vi "Teleop.vi"(10 "Match Info":T2={"Autonomous Elapsed Seconds"=0.0, "TeleOp Elapsed Seconds"=0.0, "Disabled Elapsed Seconds"=0.0, "Visited Autonomous"=FALSE, "Visited TeleOp"=FALSE, "Visited Disabled"=FALSE, "Autonomous Settings"={"Autonomous Style"=enum."Independent", "VI Refnum"=refnum}}, 11 "Call Context":T3) -> ()   [LabVIEW 2016]
doc: "This VI is called for each TeleOp packet received from the DS where the robot is not disabled. It is often used to read from the joysticks and update I/O or to update setpoints for timed control loops. It should complete and return within 20 milliseconds or it may miss DS packets."
uses:
  <vilib>/Rock Robotics/WPI/DriverStation/WPI_DriverStationDerivedRobotMode.ctl
  <vilib>/Rock Robotics/WPI/DriverStation/WPI_DriverStationMatch Info.ctl
  Robot Global Data.vi
  <vilib>/Rock Robotics/WPI/Utilities/WPI_GetSetVariantRefNum.vi
  <vilib>/addons/control/pid/pid.llb/PID (DBL).vi
  <vilib>/addons/control/pid/NI_PID_pid.lvlib
panel:
  in  "output range":cluster{"output high":dbl, "output low":dbl}={"output high"=100.0, "output low"=-100.0} {"output low" format="%.2f"; "output high" format="%.2f"}
  in  "PID gains":T1={"proportional gain (Kc)"=1.0, "integral time (Ti, min)"=0.01, "derivative time (Td, min)"=0.0} {"derivative time (Td, min)" format="%.3f"; "integral time (Ti, min)" format="%.3f"; "proportional gain (Kc)" format="%.3f"}
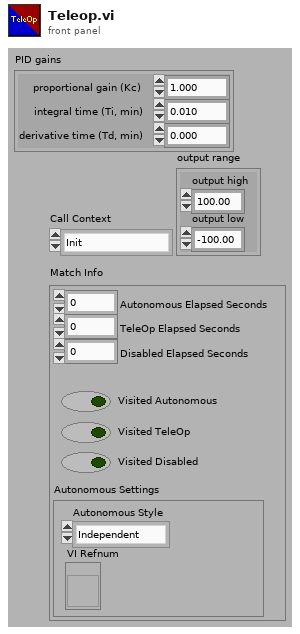
[diagram p1: front panel]
types:
  T1 = cluster{"proportional gain (Kc)":dbl, "integral time (Ti, min)":dbl, "derivative time (Td, min)":dbl}
  T2 = typedef "WPI_DriverStationMatch Info.ctl" = cluster{"Autonomous Elapsed Seconds":dbl, "TeleOp Elapsed Seconds":dbl, "Disabled Elapsed Seconds":dbl, "Visited Autonomous":bool, "Visited TeleOp":bool, "Visited Disabled":bool, "Autonomous Settings":cluster{"Autonomous Style":enum16{"Iterative", "Independent"}, "VI Refnum":refnum<vi>}}
  T3 = typedef "WPI_DriverStationDerivedRobotMode.ctl" = enum16{"Init", "Execute", "Stop"}
  T4 = typedef "WPI_RobotDriveDevRef.ctl" = cluster{"DevStatus":errorcluster, "Motors[]":T5[], "Square Inputs":bool, "Max Output":dbl}
  T5 = typedef "WPI_MotorControlDeviceRef.ctl" = cluster{"DeviceStatus":errorcluster, "Type":T6, "PWM":cluster{"PWM Channel":T7, "DeadBand":T8}, "CAN":cluster{"Device Number":u8, "SetOutput VI Ref":variant, "GetOutput VI Ref":variant, "Enable VI Ref":variant, "Disable VI Ref":variant, "Data":variant}, "Invert":bool}
  T6 = typedef "WPI_MotorControlType.ctl" = enum16{"PWM", "CAN"}
  T7 = typedef "FPGA_DIOPWMChannel.ctl" = enum8{"PWM 0", "PWM 1", "PWM 2", "PWM 3", "PWM 4", "PWM 5", "PWM 6", "PWM 7", "PWM 8", "PWM 9", "PWM MXP 0", "PWM MXP 1", "PWM MXP 2", "PWM MXP 3", "PWM MXP 4", "PWM MXP 5", "PWM MXP 6", "PWM MXP 7", "PWM MXP 8", "PWM MXP 9", "Invalid"}
  T8 = typedef "WPI_PWMDeadband.ctl" = cluster{"Name":string, "maxPositivePwm":i32, "minPositivePwm":i32, "centerPwm":i32, "maxNegativePwm":i32, "minNegativePwm":i32, "angularRange":u16}
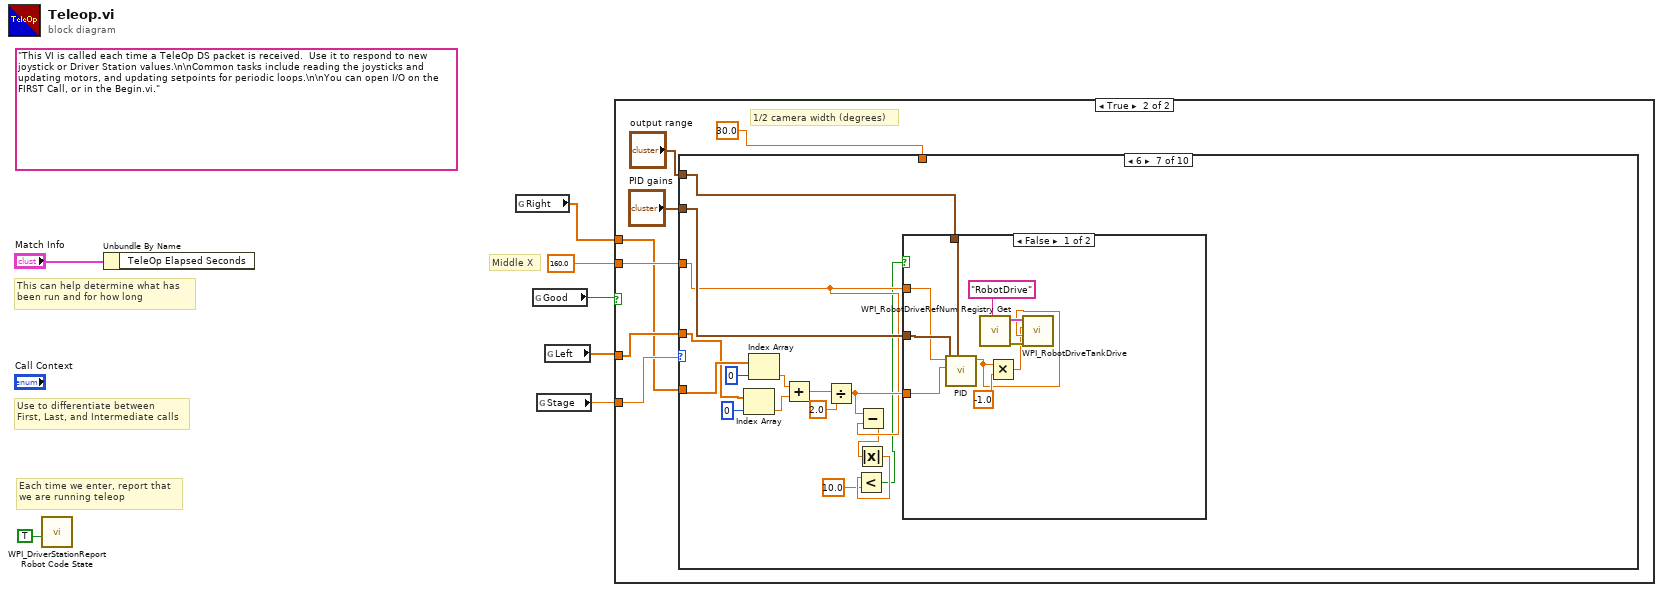
[diagram p0: block diagram]
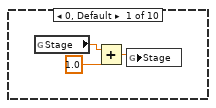
[diagram p3: hidden frame]
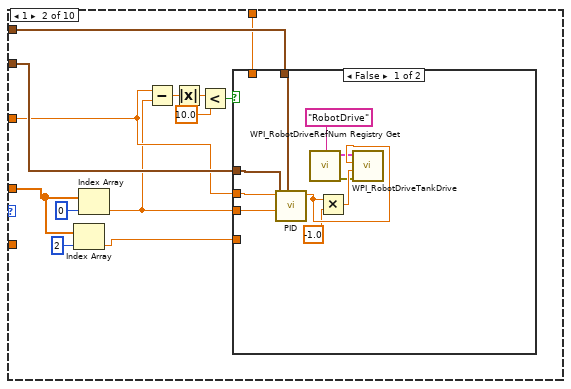
[diagram p4: hidden frame]
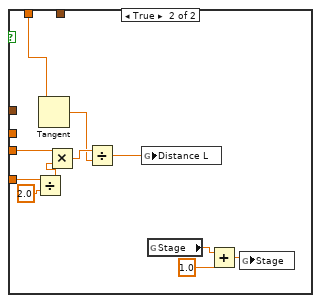
[diagram p5: hidden frame]
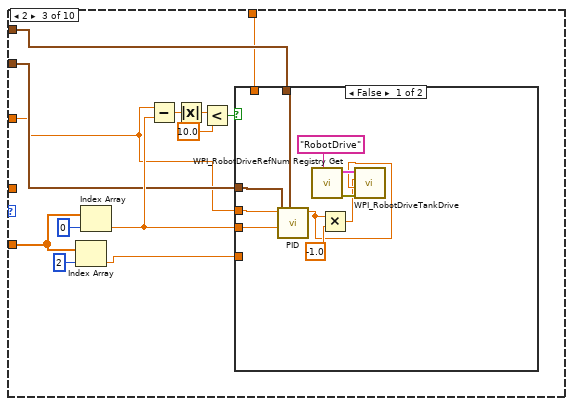
[diagram p6: hidden frame]
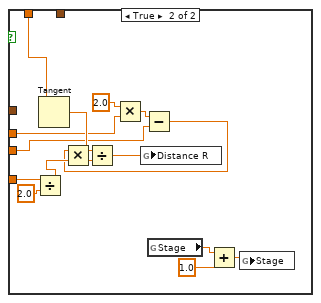
[diagram p7: hidden frame]
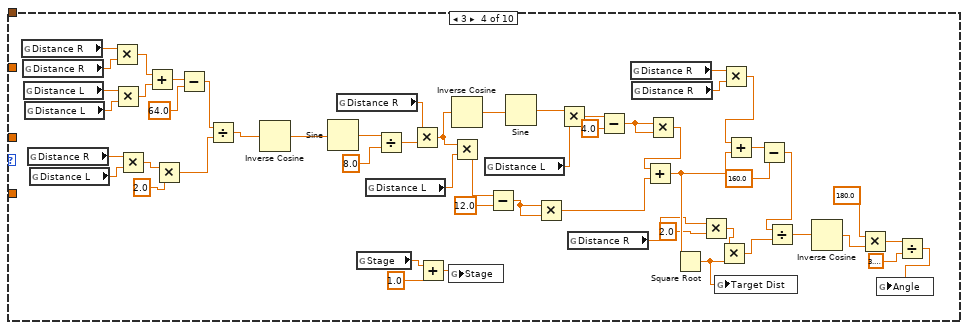
[diagram p8: hidden frame]
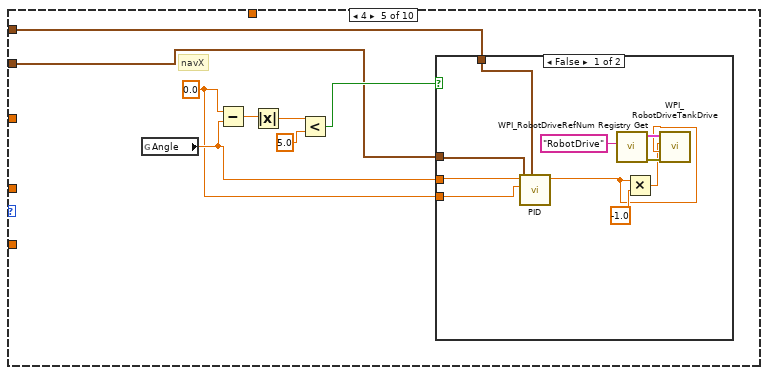
[diagram p9: hidden frame]
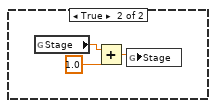
[diagram p10: hidden frame]
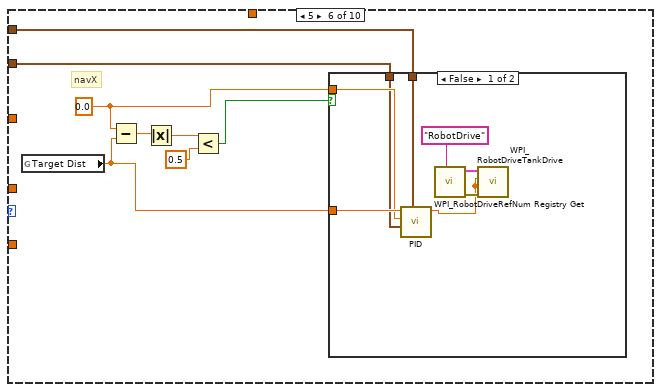
[diagram p11: hidden frame]
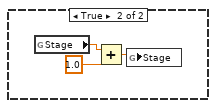
[diagram p12: hidden frame]
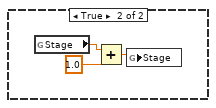
[diagram p13: hidden frame]
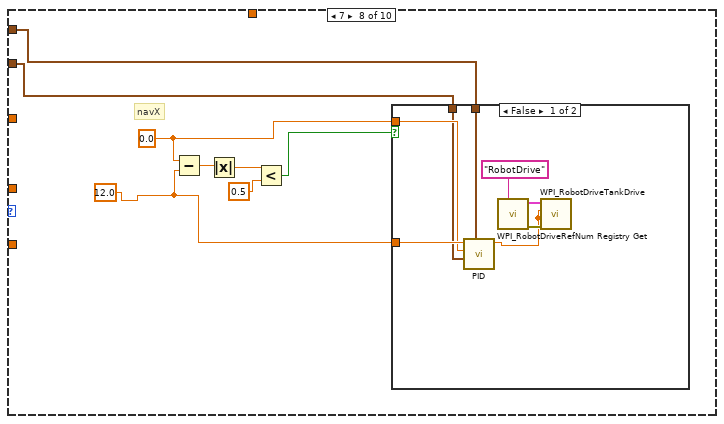
[diagram p14: hidden frame]
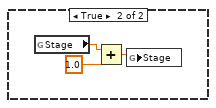
[diagram p15: hidden frame]
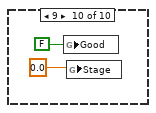
[diagram p17: hidden frame]
diagram:
  (unwired) "This VI is called each time a TeleOp DS packet is received.  Use it to respond to new joystick or Driver Station values.\n\nCommon tasks include reading the joysticks and updating motors, and updating setpoints for periodic loops.\n\nYou can open I/O on the FIRST Call, or in the Begin.vi."
  # "Middle X"
  # "Each time we enter, report that\nwe are running teleop"
  # "Use to differentiate between\nFirst, Last, and Intermediate calls"
  # "This can help determine what has\nbeen run and for how long"
  n1 = call <vilib>:"WPI_DriverStationReport Robot Code State.vi"("TeleOp"=TRUE ("Autonomous")) -> ()  [unwired: 10 in, 1 out]
  n2 = Unbundle By Name("Match Info") -> ()  [unwired: 1 out]
  n3 = global read "Robot Global Data.vi" "Right"() -> (w4:dbl[])
  n4 = global read "Robot Global Data.vi" "Good"() -> (w3:bool)
  n5 = global read "Robot Global Data.vi" "Stage"() -> (w2:dbl)
  n6 = global read "Robot Global Data.vi" "Left"() -> (w5:dbl[])
  n7 = case shown="True" w3 {
    tunnel: w4 -> [_ w8]
    tunnel: w5 -> [_ w13]
    tunnel: w2 -> [_ w14]
    tunnel: 160.0 ("setpoint") -> [_ w12]
    frame False {
    }
    frame True {
      # "1/2 camera width (degrees)"
      n8 = case shown="6" w14 {
        tunnel: w13 -> [_ w20 _ _ _ _ w194 _ _ _]
        tunnel: w12 -> [_ w27 w54 _ _ _ w188 _ _ _]
        tunnel: "PID gains" -> [_ w29 w55 _ w145 w166 w196 w215 _ _]
        tunnel: "output range" -> [_ w28 w56 _ w144 w165 w195 w214 _ _]
        tunnel: 30.0 -> [_ w21 w52 _ _ _ _ _ _ _]
        tunnel: w8 -> [_ _ w53 _ _ _ w197 _ _ _]
        frame 0, Default {
          n9 = global read "Robot Global Data.vi" "Stage"() -> (w17:dbl)
          n10 = Add(x=w17, y=1.0) -> (x+y=w15:dbl)
          n11 = global write "Robot Global Data.vi" "Stage"(w15) -> ()
        }
        frame 1 {
          n12 = Index Array(array=w20, index=2) -> (element=w18:dbl)
          n13 = Index Array(array=w20, index=0) -> (element=w26:dbl)
          n14 = Subtract(x=w27, y=w26) -> (x-y=w25:dbl)
          n15 = Absolute Value(x=w25) -> (abs(x)=w24:dbl)
          n16 = Less?(x=w24, y=10.0) -> (x < y?=w22:bool)
          n17 = case shown="False" w22 {
            tunnel: w29 -> [w34 _]
            tunnel: w28 -> [w35 _]
            tunnel: w27 -> [w33 _]
            tunnel: w26 -> [w32 w45]
            tunnel: w21 -> [_ w48]
            tunnel: w18 -> [_ w47]
            frame False {
              n18 = call-poly <vilib>:"PID.vi"("output range"=w35, "PID gains"=w34, "process variable"=w32, "setpoint"=w33) -> ("output"=w40:dbl)  [unwired: 6 in, 1 out]
              n19 = call <vilib>:"WPI_RobotDriveRefNum Registry Get.vi"("refnum name"="RobotDrive") -> ("error out"=w36:errorcluster, "RobotDriveDevRef"=w37:T4)  [unwired: 9 in]
              n20 = Multiply(x=w40, y=-1.0) -> (x*y=w39:dbl)
              n21 = call <vilib>:"WPI_RobotDriveTankDrive.vi"("error in (no error)"=w36, "Right axis value"=w39, "Left axis value"=w40, "RobotDriveDevRef"=w37) -> ()  [unwired: 5 in, 3 out]
            }
            frame True {
              n22 = Divide(x=w47, y=2.0) -> (x/y=w44:dbl)
              n23 = Tangent(1:w48) -> (0:w42:dbl)
              n24 = Multiply(x=w45, y=w44) -> (x*y=w43:dbl)
              n25 = Divide(x=w43, y=w42) -> (x/y=w41:dbl)
              n26 = global write "Robot Global Data.vi" "Distance L"(w41) -> ()
              n27 = global read "Robot Global Data.vi" "Stage"() -> (w51:dbl)
              n28 = Add(x=w51, y=1.0) -> (x+y=w49:dbl)
              n29 = global write "Robot Global Data.vi" "Stage"(w49) -> ()
            }
          }
        }
        frame 2 {
          n30 = Index Array(array=w53, index=2) -> (element=w57:dbl)
          n31 = Index Array(array=w53, index=0) -> (element=w63:dbl)
          n32 = Subtract(x=w54, y=w63) -> (x-y=w62:dbl)
          n33 = Absolute Value(x=w62) -> (abs(x)=w61:dbl)
          n34 = Less?(x=w61, y=10.0) -> (x < y?=w59:bool)
          n35 = case shown="False" w59 {
            tunnel: w55 -> [w70 _]
            tunnel: w56 -> [w71 _]
            tunnel: w54 -> [w69 w76]
            tunnel: w63 -> [w68 w77]
            tunnel: w52 -> [_ w86]
            tunnel: w57 -> [_ w85]
            frame False {
              n36 = call-poly <vilib>:"PID.vi"("output range"=w71, "PID gains"=w70, "process variable"=w68, "setpoint"=w69) -> ("output"=w67:dbl)  [unwired: 6 in, 1 out]
              n37 = call <vilib>:"WPI_RobotDriveRefNum Registry Get.vi"("refnum name"="RobotDrive") -> ("error out"=w72:errorcluster, "RobotDriveDevRef"=w73:T4)  [unwired: 9 in]
              n38 = Multiply(x=w67, y=-1.0) -> (x*y=w66:dbl)
              n39 = call <vilib>:"WPI_RobotDriveTankDrive.vi"("error in (no error)"=w72, "Right axis value"=w67, "Left axis value"=w66, "RobotDriveDevRef"=w73) -> ()  [unwired: 5 in, 3 out]
            }
            frame True {
              n40 = Divide(x=w85, y=2.0) -> (x/y=w83:dbl)
              n41 = Tangent(1:w86) -> (0:w81:dbl)
              n42 = Multiply(x=2.0, y=w76) -> (x*y=w78:dbl)
              n43 = Subtract(x=w78, y=w77) -> (x-y=w75:dbl)
              n44 = Multiply(x=w75, y=w83) -> (x*y=w82:dbl)
              n45 = Divide(x=w82, y=w81) -> (x/y=w80:dbl)
              n46 = global write "Robot Global Data.vi" "Distance R"(w80) -> ()
              n47 = global read "Robot Global Data.vi" "Stage"() -> (w89:dbl)
              n48 = Add(x=w89, y=1.0) -> (x+y=w87:dbl)
              n49 = global write "Robot Global Data.vi" "Stage"(w87) -> ()
            }
          }
        }
        frame 3 {
          n50 = global read "Robot Global Data.vi" "Distance R"() -> (w143:dbl)
          n51 = global read "Robot Global Data.vi" "Distance R"() -> (w142:dbl)
          n52 = global read "Robot Global Data.vi" "Distance L"() -> (w141:dbl)
          n53 = global read "Robot Global Data.vi" "Distance L"() -> (w140:dbl)
          n54 = global read "Robot Global Data.vi" "Distance R"() -> (w135:dbl)
          n55 = global read "Robot Global Data.vi" "Distance L"() -> (w134:dbl)
          n56 = Multiply(x=w143, y=w142) -> (x*y=w138:dbl)
          n57 = Multiply(x=w141, y=w140) -> (x*y=w139:dbl)
          n58 = Multiply(x=w135, y=w134) -> (x*y=w133:dbl)
          n59 = Add(x=w138, y=w139) -> (x+y=w137:dbl)
          n60 = Multiply(x=w133, y=2.0) -> (x*y=w130:dbl)
          n61 = Subtract(x=w137, y=64.0) -> (x-y=w131:dbl)
          n62 = Divide(x=w131, y=w130) -> (x/y=w129:dbl)
          n63 = Inverse Cosine(1:w129) -> (0:w128:dbl)
          n64 = Sine(x=w128) -> (sin(x)=w127:dbl)
          n65 = global read "Robot Global Data.vi" "Distance R"() -> (w124:dbl)
          n66 = global read "Robot Global Data.vi" "Stage"() -> (w92:dbl)
          n67 = global read "Robot Global Data.vi" "Distance L"() -> (w123:dbl)
          n68 = Divide(x=w127, y=8.0) -> (x/y=w125:dbl)
          n69 = Multiply(x=w124, y=w125) -> (x*y=w122:dbl)
          n70 = Add(x=w92, y=1.0) -> (x+y=w90:dbl)
          n71 = global write "Robot Global Data.vi" "Stage"(w90) -> ()
          n72 = Inverse Cosine(1:w122) -> (0:w121:dbl)
          n73 = Multiply(x=w122, y=w123) -> (x*y=w118:dbl)
          n74 = global read "Robot Global Data.vi" "Distance L"() -> (w119:dbl)
          n75 = Subtract(x=w118, y=12.0) -> (x-y=w114:dbl)
          n76 = Sine(x=w121) -> (sin(x)=w120:dbl)
          n77 = Multiply(x=w114, y=w114) -> (x*y=w111:dbl)
          n78 = Multiply(x=w120, y=w119) -> (x*y=w116:dbl)
          n79 = global read "Robot Global Data.vi" "Distance R"() -> (w102:dbl)
          n80 = Subtract(x=w116, y=4.0) -> (x-y=w113:dbl)
          n81 = global read "Robot Global Data.vi" "Distance R"() -> (w110:dbl)
          n82 = global read "Robot Global Data.vi" "Distance R"() -> (w109:dbl)
          n83 = Multiply(x=w113, y=w113) -> (x*y=w112:dbl)
          n84 = Add(x=w112, y=w111) -> (x+y=w108:dbl)
          n85 = Square Root(x=w108) -> (sqrt(x)=w94:dbl)
          n86 = Multiply(x=w102, y=2.0) -> (x*y=w104:dbl)
          n87 = global write "Robot Global Data.vi" "Target Dist"(w94) -> ()
          n88 = Multiply(x=w104, y=w94) -> (x*y=w100:dbl)
          n89 = Multiply(x=w110, y=w109) -> (x*y=w107:dbl)
          n90 = Add(x=w107, y=w108) -> (x+y=w106:dbl)
          n91 = Subtract(x=w106, y=160.0) -> (x-y=w101:dbl)
          n92 = Divide(x=w101, y=w100) -> (x/y=w99:dbl)
          n93 = Inverse Cosine(1:w99) -> (0:w98:dbl)
          n94 = Multiply(x=180.0, y=w98) -> (x*y=w96:dbl)
          n95 = Divide(x=w96, y=3.141592653589793) -> (x/y=w93:dbl)
          n96 = global write "Robot Global Data.vi" "Angle"(w93) -> ()
        }
        frame 4 {
          w146 = 0.0
          # "navX"
          n97 = global read "Robot Global Data.vi" "Angle"() -> (w147:dbl)
          n98 = Subtract(x=w146, y=w147) -> (x-y=w151:dbl)
          n99 = Absolute Value(x=w151) -> (abs(x)=w150:dbl)
          n100 = Less?(x=w150, y=5.0) -> (x < y?=w148:bool)
          n101 = case shown="False" w148 {
            tunnel: w145 -> [w158 _]
            tunnel: w144 -> [w153 _]
            tunnel: w147 -> [w157 _]
            tunnel: w146 -> [w154 _]
            frame False {
              n102 = call-poly <vilib>:"PID.vi"("output range"=w153, "PID gains"=w158, "process variable"=w154, "setpoint"=w157) -> ("output"=w156:dbl)  [unwired: 6 in, 1 out]
              n103 = call <vilib>:"WPI_RobotDriveRefNum Registry Get.vi"("refnum name"="RobotDrive") -> ("error out"=w159:errorcluster, "RobotDriveDevRef"=w160:T4)  [unwired: 9 in]
              n104 = Multiply(x=w156, y=-1.0) -> (x*y=w155:dbl)
              n105 = call <vilib>:"WPI_RobotDriveTankDrive.vi"("error in (no error)"=w159, "Right axis value"=w156, "Left axis value"=w155, "RobotDriveDevRef"=w160) -> ()  [unwired: 5 in, 3 out]
            }
            frame True {
              n106 = global read "Robot Global Data.vi" "Stage"() -> (w164:dbl)
              n107 = Add(x=w164, y=1.0) -> (x+y=w162:dbl)
              n108 = global write "Robot Global Data.vi" "Stage"(w162) -> ()
            }
          }
        }
        frame 5 {
          w167 = 0.0
          # "navX"
          n109 = global read "Robot Global Data.vi" "Target Dist"() -> (w168:dbl)
          n110 = Subtract(x=w167, y=w168) -> (x-y=w172:dbl)
          n111 = Absolute Value(x=w172) -> (abs(x)=w171:dbl)
          n112 = Less?(x=w171, y=0.5) -> (x < y?=w169:bool)
          n113 = case shown="False" w169 {
            tunnel: w168 -> [w178 _]
            tunnel: w167 -> [w177 _]
            tunnel: w166 -> [w176 _]
            tunnel: w165 -> [w175 _]
            frame False {
              n114 = call-poly <vilib>:"PID.vi"("output range"=w175, "PID gains"=w176, "process variable"=w177, "setpoint"=w178) -> ("output"=w174:dbl)  [unwired: 6 in, 1 out]
              n115 = call <vilib>:"WPI_RobotDriveRefNum Registry Get.vi"("refnum name"="RobotDrive") -> ("error out"=w179:errorcluster, "RobotDriveDevRef"=w180:T4)  [unwired: 9 in]
              n116 = call <vilib>:"WPI_RobotDriveTankDrive.vi"("error in (no error)"=w179, "Right axis value"=w174, "Left axis value"=w174, "RobotDriveDevRef"=w180) -> ()  [unwired: 5 in, 3 out]
            }
            frame True {
              n117 = global read "Robot Global Data.vi" "Stage"() -> (w183:dbl)
              n118 = Add(x=w183, y=1.0) -> (x+y=w181:dbl)
              n119 = global write "Robot Global Data.vi" "Stage"(w181) -> ()
            }
          }
        }
        frame 6 {
          n120 = Index Array(array=w194, index=0) -> (element=w192:dbl)
          n121 = Index Array(array=w197, index=0) -> (element=w193:dbl)
          n122 = Add(x=w193, y=w192) -> (x+y=w191:dbl)
          n123 = Divide(x=w191, y=2.0) -> (x/y=w189:dbl)
          n124 = Subtract(x=w189, y=w188) -> (x-y=w187:dbl)
          n125 = Absolute Value(x=w187) -> (abs(x)=w186:dbl)
          n126 = Less?(x=w186, y=10.0) -> (x < y?=w184:bool)
          n127 = case shown="False" w184 {
            tunnel: w196 -> [w205 _]
            tunnel: w195 -> [w206 _]
            tunnel: w189 -> [w202 _]
            tunnel: w188 -> [w201 _]
            frame False {
              n128 = call-poly <vilib>:"PID.vi"("output range"=w206, "PID gains"=w205, "process variable"=w202, "setpoint"=w201) -> ("output"=w204:dbl)  [unwired: 6 in, 1 out]
              n129 = call <vilib>:"WPI_RobotDriveRefNum Registry Get.vi"("refnum name"="RobotDrive") -> ("error out"=w207:errorcluster, "RobotDriveDevRef"=w208:T4)  [unwired: 9 in]
              n130 = Multiply(x=w204, y=-1.0) -> (x*y=w203:dbl)
              n131 = call <vilib>:"WPI_RobotDriveTankDrive.vi"("error in (no error)"=w207, "Right axis value"=w204, "Left axis value"=w203, "RobotDriveDevRef"=w208) -> ()  [unwired: 5 in, 3 out]
            }
            frame True {
              n132 = global read "Robot Global Data.vi" "Stage"() -> (w212:dbl)
              n133 = Add(x=w212, y=1.0) -> (x+y=w210:dbl)
              n134 = global write "Robot Global Data.vi" "Stage"(w210) -> ()
            }
          }
        }
        frame 7 {
          w213 = 12.0
          w216 = 0.0
          # "navX"
          n135 = Subtract(x=w216, y=w213) -> (x-y=w220:dbl)
          n136 = Absolute Value(x=w220) -> (abs(x)=w219:dbl)
          n137 = Less?(x=w219, y=0.5) -> (x < y?=w217:bool)
          n138 = case shown="False" w217 {
            tunnel: w213 -> [w226 _]
            tunnel: w216 -> [w225 _]
            tunnel: w215 -> [w224 _]
            tunnel: w214 -> [w223 _]
            frame False {
              n139 = call-poly <vilib>:"PID.vi"("output range"=w223, "PID gains"=w224, "process variable"=w225, "setpoint"=w226) -> ("output"=w222:dbl)  [unwired: 6 in, 1 out]
              n140 = call <vilib>:"WPI_RobotDriveRefNum Registry Get.vi"("refnum name"="RobotDrive") -> ("error out"=w227:errorcluster, "RobotDriveDevRef"=w228:T4)  [unwired: 9 in]
              n141 = call <vilib>:"WPI_RobotDriveTankDrive.vi"("error in (no error)"=w227, "Right axis value"=w222, "Left axis value"=w222, "RobotDriveDevRef"=w228) -> ()  [unwired: 5 in, 3 out]
            }
            frame True {
              n142 = global read "Robot Global Data.vi" "Stage"() -> (w231:dbl)
              n143 = Add(x=w231, y=1.0) -> (x+y=w229:dbl)
              n144 = global write "Robot Global Data.vi" "Stage"(w229) -> ()
            }
          }
        }
        frame 8 {
          # "Active Mechanism"
        }
        frame 9 {
          n145 = global write "Robot Global Data.vi" "Good"(FALSE) -> ()
          n146 = global write "Robot Global Data.vi" "Stage"(0.0) -> ()
        }
      }
    }
  }
